vi "DriveForDistance.vi"(10 "Speed":dbl, 11 "Distance":dbl) -> ()   [LabVIEW 2017]
uses:
  RoutineData.vi
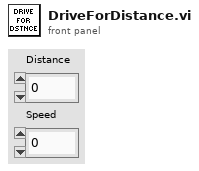
[diagram p1: front panel]
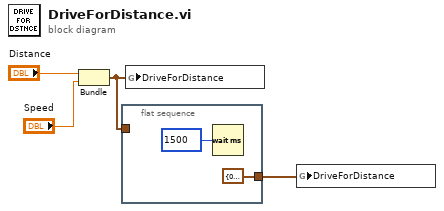
[diagram p0: block diagram]
diagram:
  n1 = Bundle("Distance"="Distance", "Speed"="Speed") -> (w2:cluster{"Distance":dbl, "Speed":dbl})  [unwired: 1 in]
  n2 = flat-sequence {
    tunnel: w2 -> [_]
    tunnel: [cluster{"Distance":dbl, "Speed":dbl} {"Distance"=0.0, "Speed"=0.0} ("output cluster")] -> w1
    frame #0 {
      n3 = Wait (ms)(milliseconds to wait=u32 1500) -> ()  [unwired: 1 out]
    }
  }
  n4 = global write "RoutineData.vi" "DriveForDistance"(w2) -> ()
  n5 = global write "RoutineData.vi" "DriveForDistance"(w1) -> ()
